vi "flow-builder.orp-dosing.vi"(7 "Proc Name":string="\n", 8 "error in":errorcluster, 9 "Unit Index":i32, 11 "Nutrition Cluster":T3 {"ORP Dosing"."MIX Limit" format="%d [s]"; "ORP Dosing"."MIX Dose" format="%d [s]"; "PH Dosing"."ACID Limit" format="%d [s]"; "PH Dosing"."BASE Limit" format="%d [s]"; "PH Dosing"."ACID Dose" format="%d [s]"; "PH Dosing"."BASE Dose" format="%d [s]"; "EC Dosing"."BETA2 Limit" format="%d [s]"; "EC Dosing"."ALFA2 Limit" format="%d [s]"; "EC Dosing"."ALFA2 Dose" format="%d [s]"; "EC Dosing"."BETA2 Dose" format="%d [s]"; "EC Dosing"."BETA1 Limit" format="%d [s]"; "EC Dosing"."ALFA1 Limit" format="%d [s]"; "EC Dosing"."ALFA1 Dose" format="%d [s]"; "EC Dosing"."BETA1 Dose" format="%d [s]"; "Main"."DailyActivityHours"."Begin Time" format="ON:    %<%H:%M>T"; "Main"."DailyActivityHours"."End Time" format="OFF:    %<%H:%M>T"; "Main"."WashTimes"."Out" format="Wash out: %d [sec]"; "Main"."WashTimes"."In" format="Wash in: %d [sec]"; "Water Dosing"."Water Limit" format="%d [s]"; "Water Dosing"."Water Dose" format="%d [s]"}) -> (0 "error out":errorcluster, 1 "WillDose?":bool, 2 "status":string, 3 "Flow out":T1[](array[typedef]))   [LabVIEW 2024]
uses:
  controls/UiNutritionPanel.ctl
  controls/UiScheduleTimestamp.ctl
  controls/UiStepBuilder.ctl
  controls/type.step-builder.ctl
  controls/enum-ntr-io-format.ctl
  io.interface.serial.vi
  <vilib>/Utility/error.llb/Trim Whitespace One-Sided.vi
  <vilib>/Utility/error.llb/Clear Errors.vi
  Polymorphics/variantCtrlIo.vi
  globals/globals-engine.vi
  util.environment.vi
  util-address-parser.vi
  util-address-builder.vi
  util.DO.ToString.vi
  Polymorphics/io.command-builder.vi
  Polymorphics/io.command-builder.DO.vi
  Polymorphics/io.command-builder.AI.vi
  Polymorphics/io.command-builder.DI.vi
  io.frame.vi
  io.visa.vi
  io.responseValidator.vi
  Polymorphics/io.command-parser.DI.vi
  Polymorphics/io.command-parser.AI.vi
panel:
  out "Dosing Tabel":cluster{"Dose Time":dbl, "Input":string}[](array[cluster])
  in  "simulator":dbl=3.0
  out "Low Range":bool
  out "Low Alarm":bool
  out "High Alarm":bool
  # "Water"
  # "EC"
  # "PH"
  # "ORP"
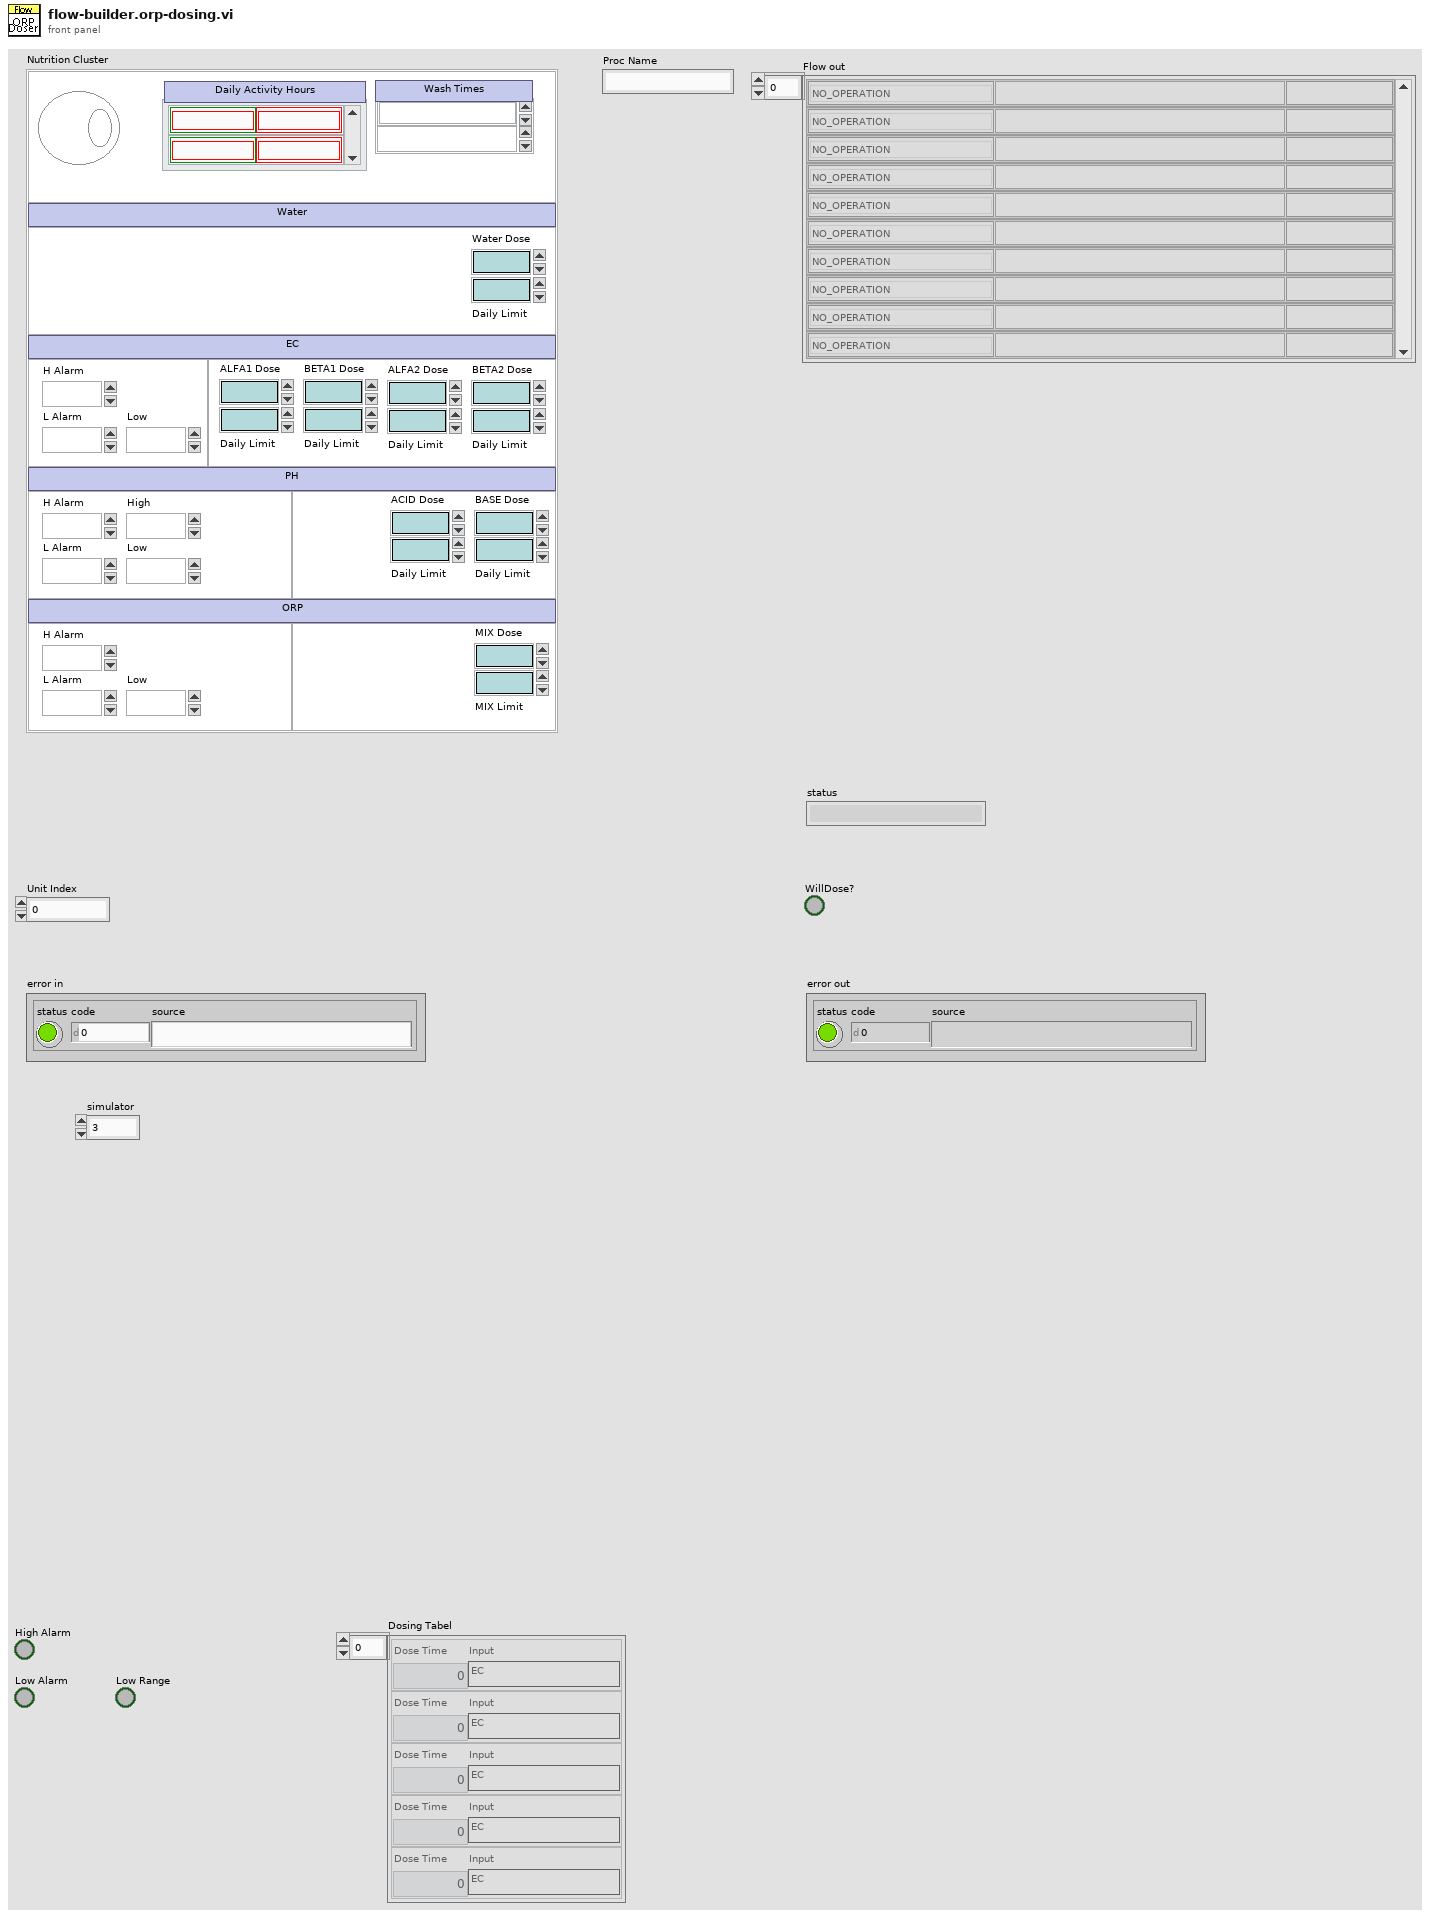
[diagram p1: front panel]
types:
  T1 = typedef "UiStepBuilder.ctl" = cluster{"Step Function":T2, "ParamString":string, "Step Label":string}
  T2 = typedef "type.step-builder.ctl" = enum16{"NO_OPERATION", "DELAY-JUMP", "DELAY", "JUMP", "COMPLETE", "SCHEDULER", "IRR-CHECK", "UNIT-CHECK", "UNIT-SAMPLE", "UNIT-DOSE", "LOG-REPORT", "LOG-MESSAGE", "IO-READ", "IO-READ-MANY", "IO-WRITE", "IO-COMPARE-OUT", "IO-COMPARE-IN", "PROC-START", "PROC-STOP", "PROC-LOAD", "PROC-IS-COMPLETED", "RECORD-MOVE", "GET-RH", "GET-UV", "GET-WD", "GET-WS", "OCS-CHECK", "OCS-RECORD"}
  T3 = typedef "UiNutritionPanel.ctl" = cluster{"Main":cluster{"Enable":bool, "WashTimes":cluster{"In":dbl, "Out":dbl}, "DailyActivityHours":cluster{"Begin Time":T4, "End Time":T4}[]}, "Water Dosing":cluster{"Water Dose":dbl, "Water Limit":dbl}, "EC Ranges":cluster{"H Alarm":dbl, "L Alarm":dbl, "Low":dbl}, "EC Dosing":cluster{"ALFA1 Dose":dbl, "ALFA1 Limit":dbl, "BETA1 Dose":dbl, "BETA1 Limit":dbl, "ALFA2 Dose":dbl, "ALFA2 Limit":dbl, "BETA2 Dose":dbl, "BETA2 Limit":dbl}, "PH Ranges":cluster{"H Alarm":dbl, "L Alarm":dbl, "High":dbl, "Low":dbl}, "PH Dosing":cluster{"ACID Dose":dbl, "ACID Limit":dbl, "BASE Dose":dbl, "BASE Limit":dbl}, "ORP Ranges":cluster{"H Alarm":dbl, "L Alarm":dbl, "Low":dbl}, "ORP Dosing":cluster{"MIX Dose":dbl, "MIX Limit":dbl}}
  T4 = typedef "UiScheduleTimestamp.ctl" = timestamp
  T5 = typedef "enum-ntr-io-format.ctl" = enum16{"UN_VLV%d", "UN_PMP%d", "UN_WL%d", "UN_PH", "UN_EC", "UN_ORP", "UN_WT", "UN_PH2", "UN_ALFA1", "UN_BETA1", "UN_ALFA2", "UN_BETA2", "UN_ACID", "UN_BASE", "UN_WATER", "UN_ORPMIX"}
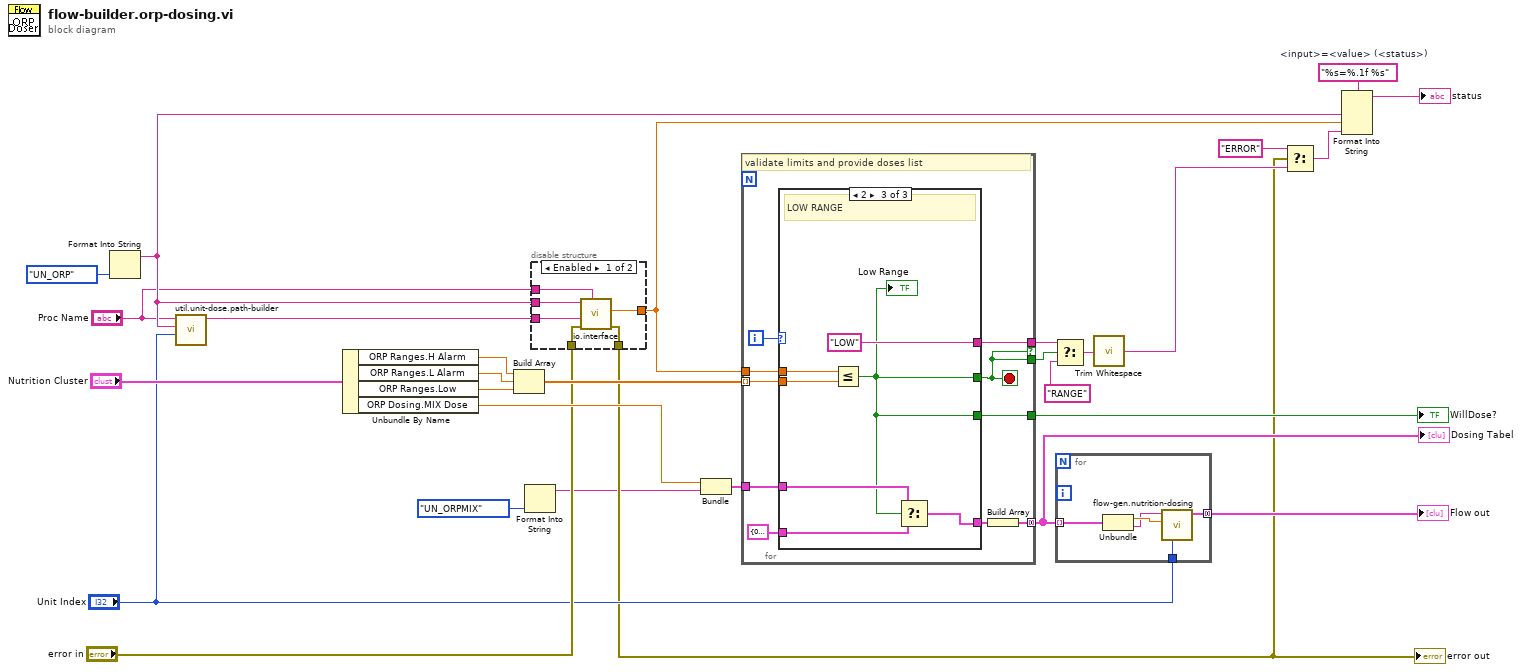
[diagram p0: block diagram]
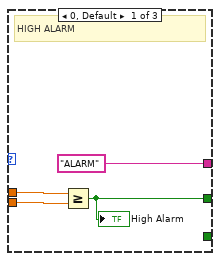
[diagram p2: hidden frame]
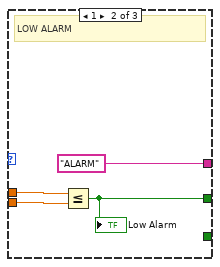
[diagram p3: hidden frame]
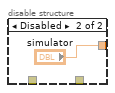
[diagram p4: hidden frame]
diagram:
  w13 = "%s=%.1f %s"  # <input>=<value> (<status>)
  n1 = Format Into String(enum-ntr-io-format."UN_ORP") -> (resulting string=w4:string)  [unwired: 3 in, 1 out]
  n2 = call "util.unit-dose.path-builder.vi"("Unit Index"="Unit Index", "Input"=w4, "Proc Name"="Proc Name") -> ("\\NUTRITION\\ORP\\ORP_U1_2024-08-16.*"=w17:string)  [unwired: 8 in]
  n3 = Unbundle By Name("Nutrition Cluster") -> ("ORP Ranges.H Alarm"=w29:dbl, "ORP Ranges.L Alarm"=w27:dbl, "ORP Ranges.Low"=w26:dbl, "ORP Dosing.MIX Dose"=w22:dbl)
  n4 = Build Array(w29, w27, w26) -> (w28:dbl[])
  n5 = Format Into String(enum-ntr-io-format."UN_ORPMIX") -> (resulting string=w2:string)  [unwired: 3 in, 1 out]
  n6 = disable-structure shown="Enabled" {
    disable-tunnel: w4 -> [w35 _]
    disable-tunnel: [w34 "simulator"] -> w12
    disable-tunnel: [w33 _] -> w6
    disable-tunnel: "error in" -> [w32 _]
    disable-tunnel: w17 -> [w31 _]
    disable-tunnel: "Proc Name" -> [w30 _]
    frame Enabled {
      n7 = call "io.interface.vi"("Caller"=w30, "error in"=w32, "record filename.* (disabled if empty)"=w31, "IO Name in"=w35) -> ("error out"=w33:errorcluster, "Value out"=w34:dbl)  [unwired: 2 in, 4 out]
    }
    frame Disabled {
    }
  }
  "error out" <- w6
  n8 = Bundle("MIX Dose"=w22, w2) -> (w21:cluster{"MIX Dose":dbl, string})  [unwired: 1 in]
  n9 = for {
    tunnel: w28 -> [w45] mode=indexing
    tunnel: [w44] -> w15 if=w42
    tunnel: w12 -> [w43]
    tunnel: [w42] -> w16
    tunnel: [w40] -> w24 mode=concatenating
    tunnel: w21 -> [w39]
    tunnel: [w37] -> w10
    i -> [w46]
    stop <- w42 stop-if-true
    # "validate limits and provide doses list"
    n10 = case shown="2" w46 {
      tunnel: w45 -> [w49 w53 w60]
      tunnel: [w47 w51 w55] -> w42
      tunnel: ["ALARM" "ALARM" "LOW"] -> w44
      tunnel: w43 -> [w48 w52 w59]
      tunnel: [_ _ w58] -> w41
      tunnel: w39 -> [_ _ w56]
      tunnel: cluster{"BETA-2":dbl, "I/O":string} {"BETA-2"=0.0, "I/O"=""} ("f") -> [_ _ w57]
      tunnel: [_ _ w55] -> w37
      frame 0, Default {
        # "HIGH ALARM"
        n11 = Greater Or Equal?(x=w48, y=w49) -> (x >= y?=w47:bool)
        "High Alarm" <- w47
      }
      frame 1 {
        # "LOW ALARM"
        n12 = Less Or Equal?(x=w52, y=w53) -> (x <= y?=w51:bool)
        "Low Alarm" <- w51
      }
      frame 2 {
        # "LOW RANGE"
        n13 = Less Or Equal?(x=w59, y=w60) -> (x <= y?=w55:bool)
        "Low Range" <- w55
        n14 = Select(t=w56, s=w55, f=w57) -> (s? t:f=w58:cluster{"BETA-2":dbl, "I/O":string})
      }
    }
    n15 = Build Array(w41) -> (w40:cluster{"BETA-2":dbl, "I/O":string}[])
  }
  "Dosing Tabel" <- w24
  "WillDose?" <- w10
  n16 = Select(t=w15, s=w16, f="RANGE") -> (s? t:f=w11:string)
  n17 = for {
    tunnel: [w66] -> w23 mode=concatenating
    tunnel: w24 -> [w65] mode=indexing
    tunnel: "Unit Index" -> [w62]
    n18 = Unbundle(w65) -> ("BETA-2"=w64:dbl, "I/O"=w63:string)
    n19 = call "flow-gen.nutrition-dosing.vi"("Unit Index"=w62, "Dosing Time"=w64, "IO Name"=w63) -> ("Flow"=w66:T1[])  [unwired: 7 in, 1 out]
  }
  "Flow out" <- w23
  n20 = call <vilib>:"Trim Whitespace.vi"("string"=w11) -> ("trimmed string"=w8:string)  [unwired: 1 in]
  n21 = Select(t="ERROR", s=w6, f=w8) -> (s? t:f=w7:string)
  n22 = Format Into String(format string=w13, w4, w12, w7) -> (resulting string=→"status":string)  [unwired: 2 in, 1 out]
